vi "live_edited.vi"() -> ()   [LabVIEW 2020]
uses:
  C:/Users/Public/Documents/Photometrics/PMQI-LabViewSamples/Examples/2018/Dependencies/PVCamNET.dll
  Dependencies/PVCamNET.dll
panel:
  out "Trigger Mode":i32
  in  "Trigger In Behaviour":string(combo)
  out "Exp. out":i32
  in  "Trigger Out Behaviour":string(combo)
  out "Boolean":bool
  in  "Scan Direction Reset":bool
  out "Scan Line Time":dbl format="%#_14g"
  in  "Scan Width":dbl
  in  "Scan Line Delay":dbl
  in  "Scan Direction":string(combo)
  in  "Scan Mode":string(combo)
  in  "Exposure Time":dbl
  in  "Live":bool
  in  "Camera Status":bool
  in  "Uninit":bool
  in  "Live stop":bool
  in  "Live start":bool
  in  "Open":bool
  # "SimpleLiveAppProgrammableScanMode.vi\n\nDescription:\nThis sample code lets the user use programmable scan\n mode in an event driven structure.\n\nSteps to run:\n1. Click \"Run\"\n2. Click \"Open\"\n3. Enter Exposure Time\n4. Select Scan Mode. \n5. Set Scan Line Delay or Scan Width\n6. Select Scan Direction\n7. Click \"Live start\"\n8. Click \"Live stop\"\n9. Click \"Close\""
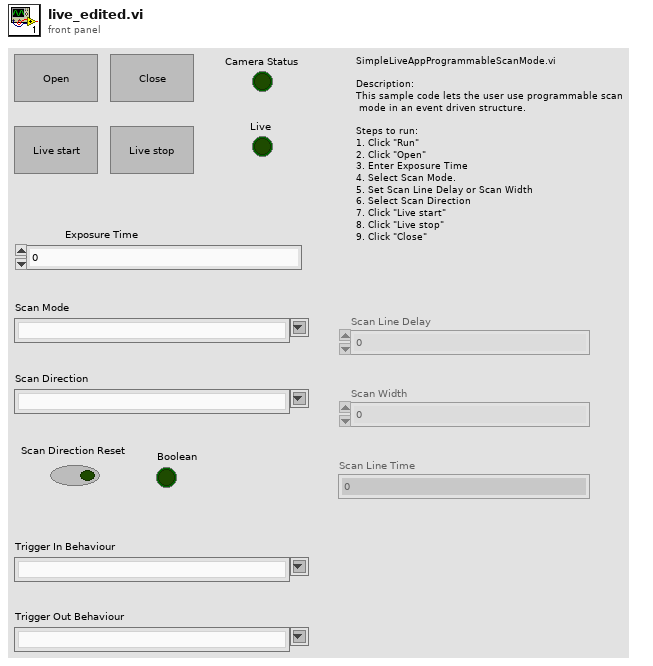
[diagram p1: front panel]
types:
  T1 = enum8{"Enabled", "Disabled", "Disabled and Grayed Out"}
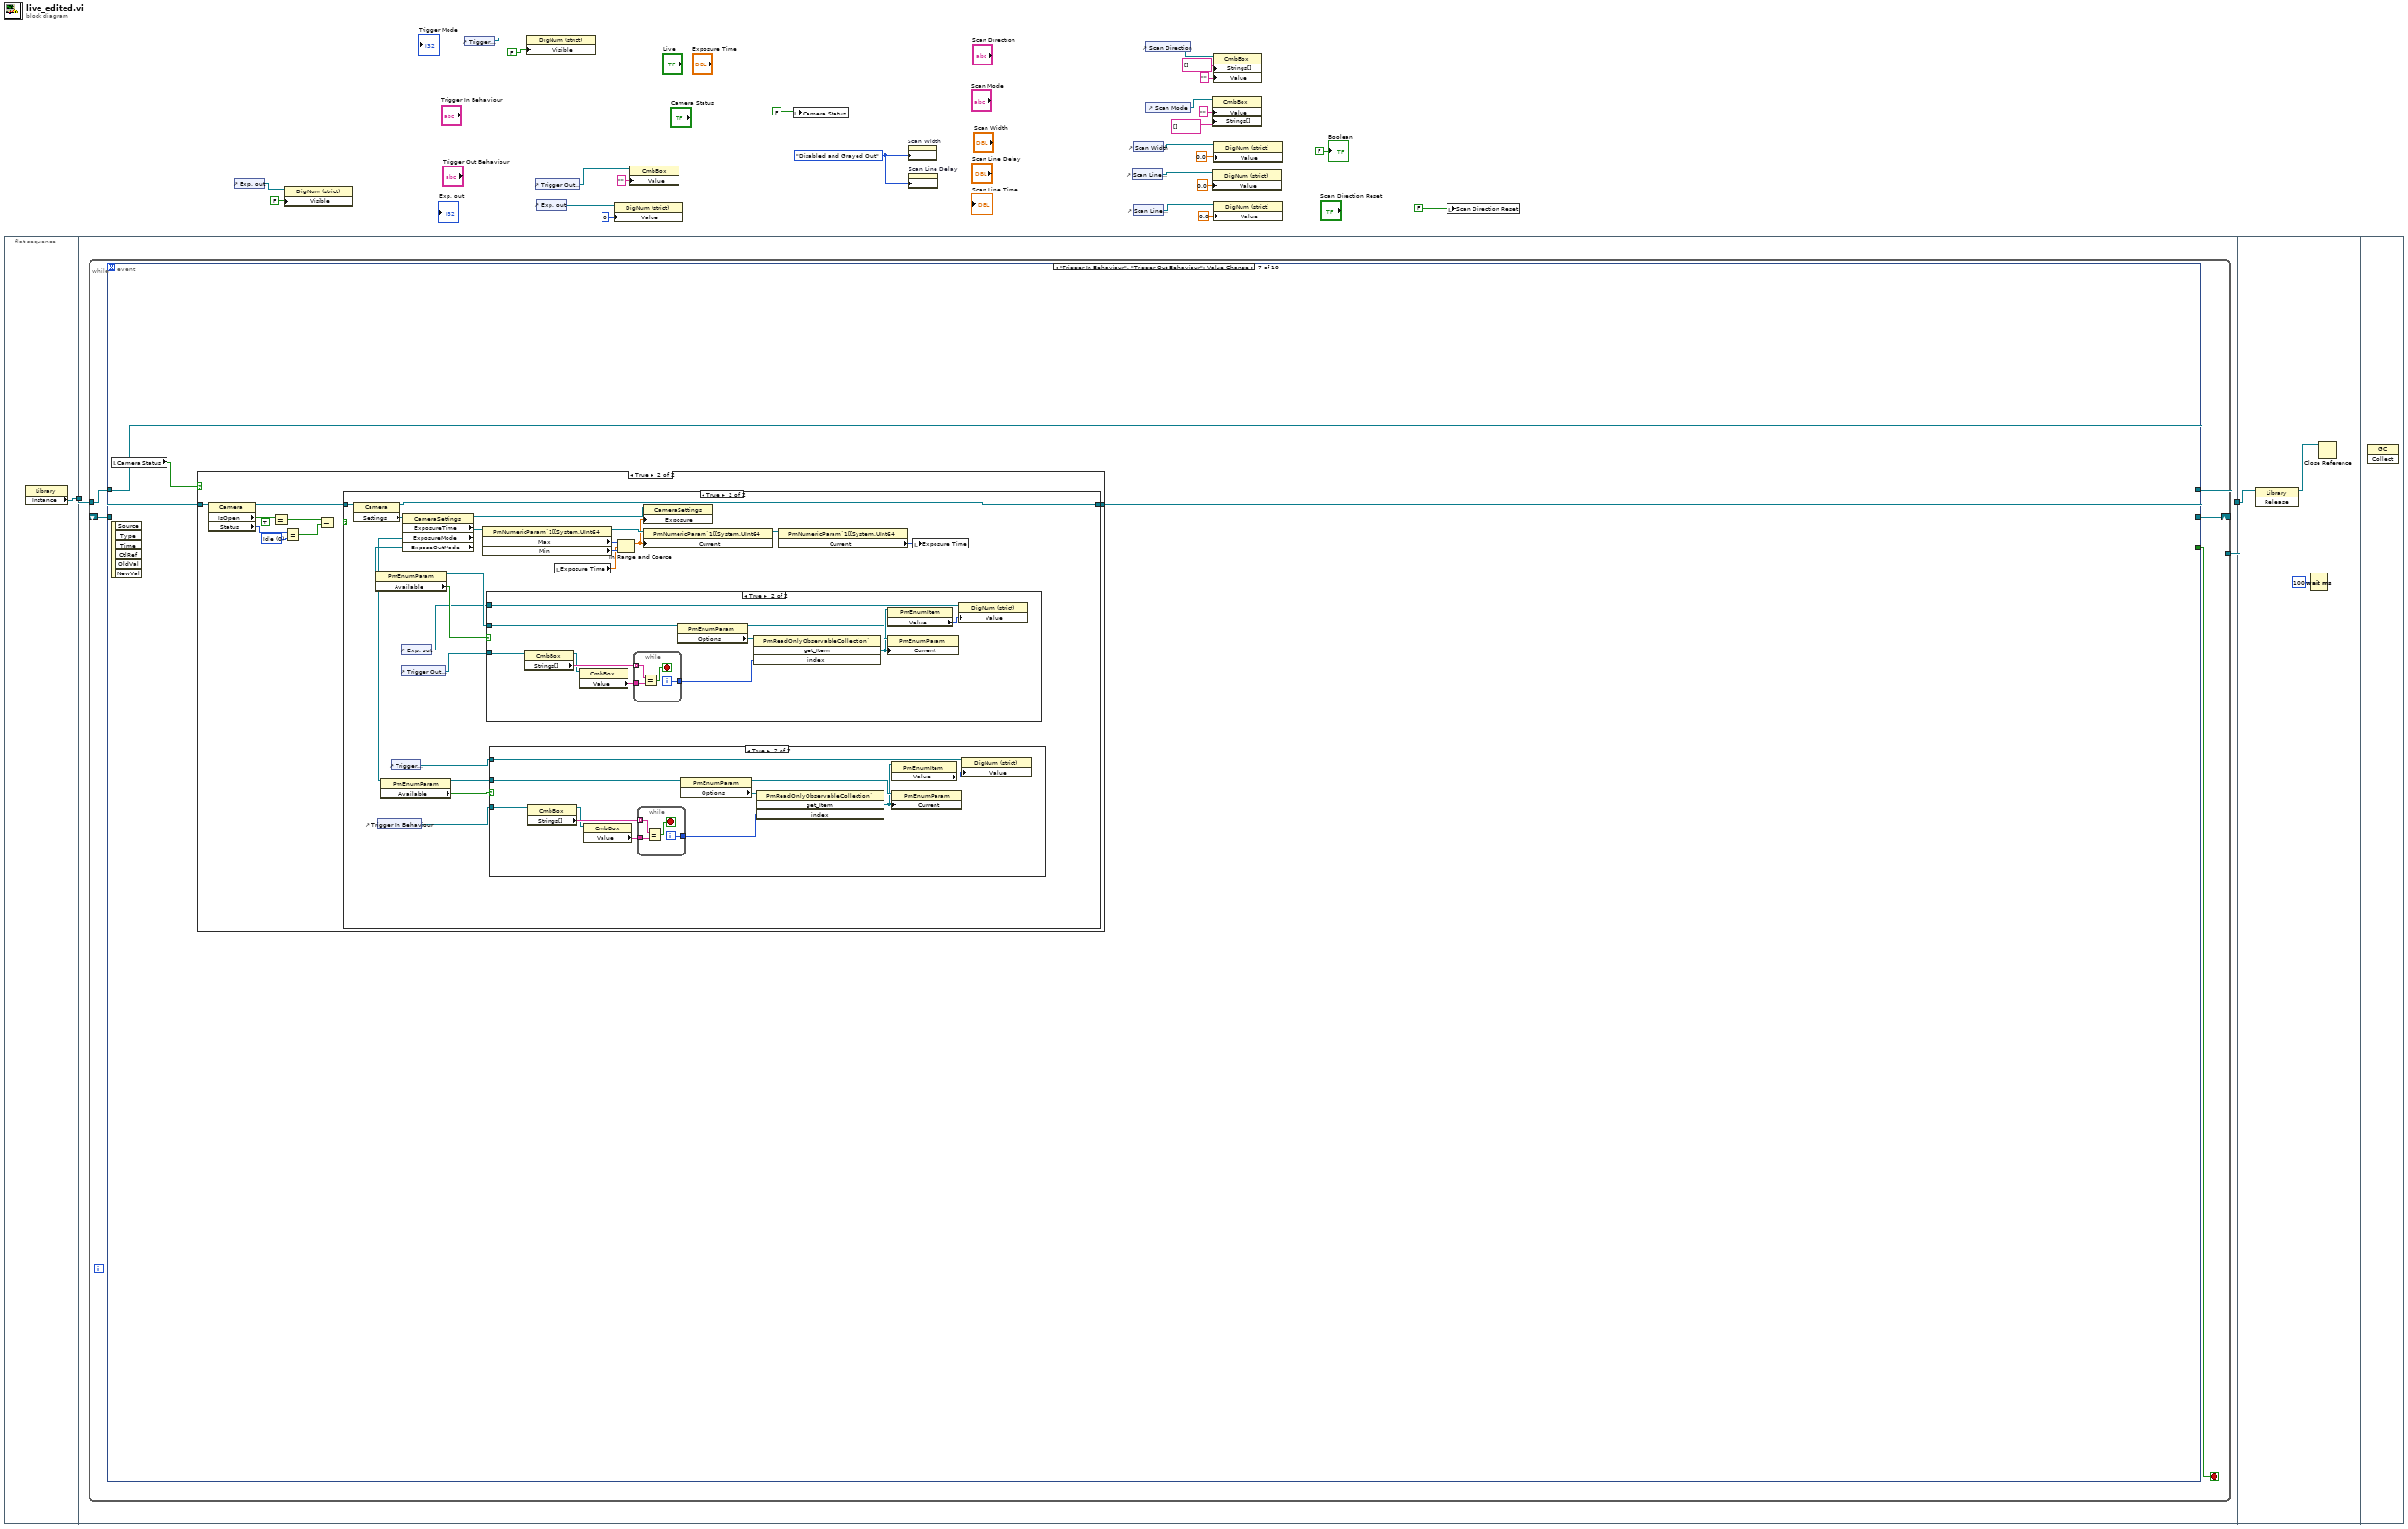
[diagram p0: block diagram]
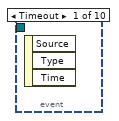
[diagram p2: hidden frame]
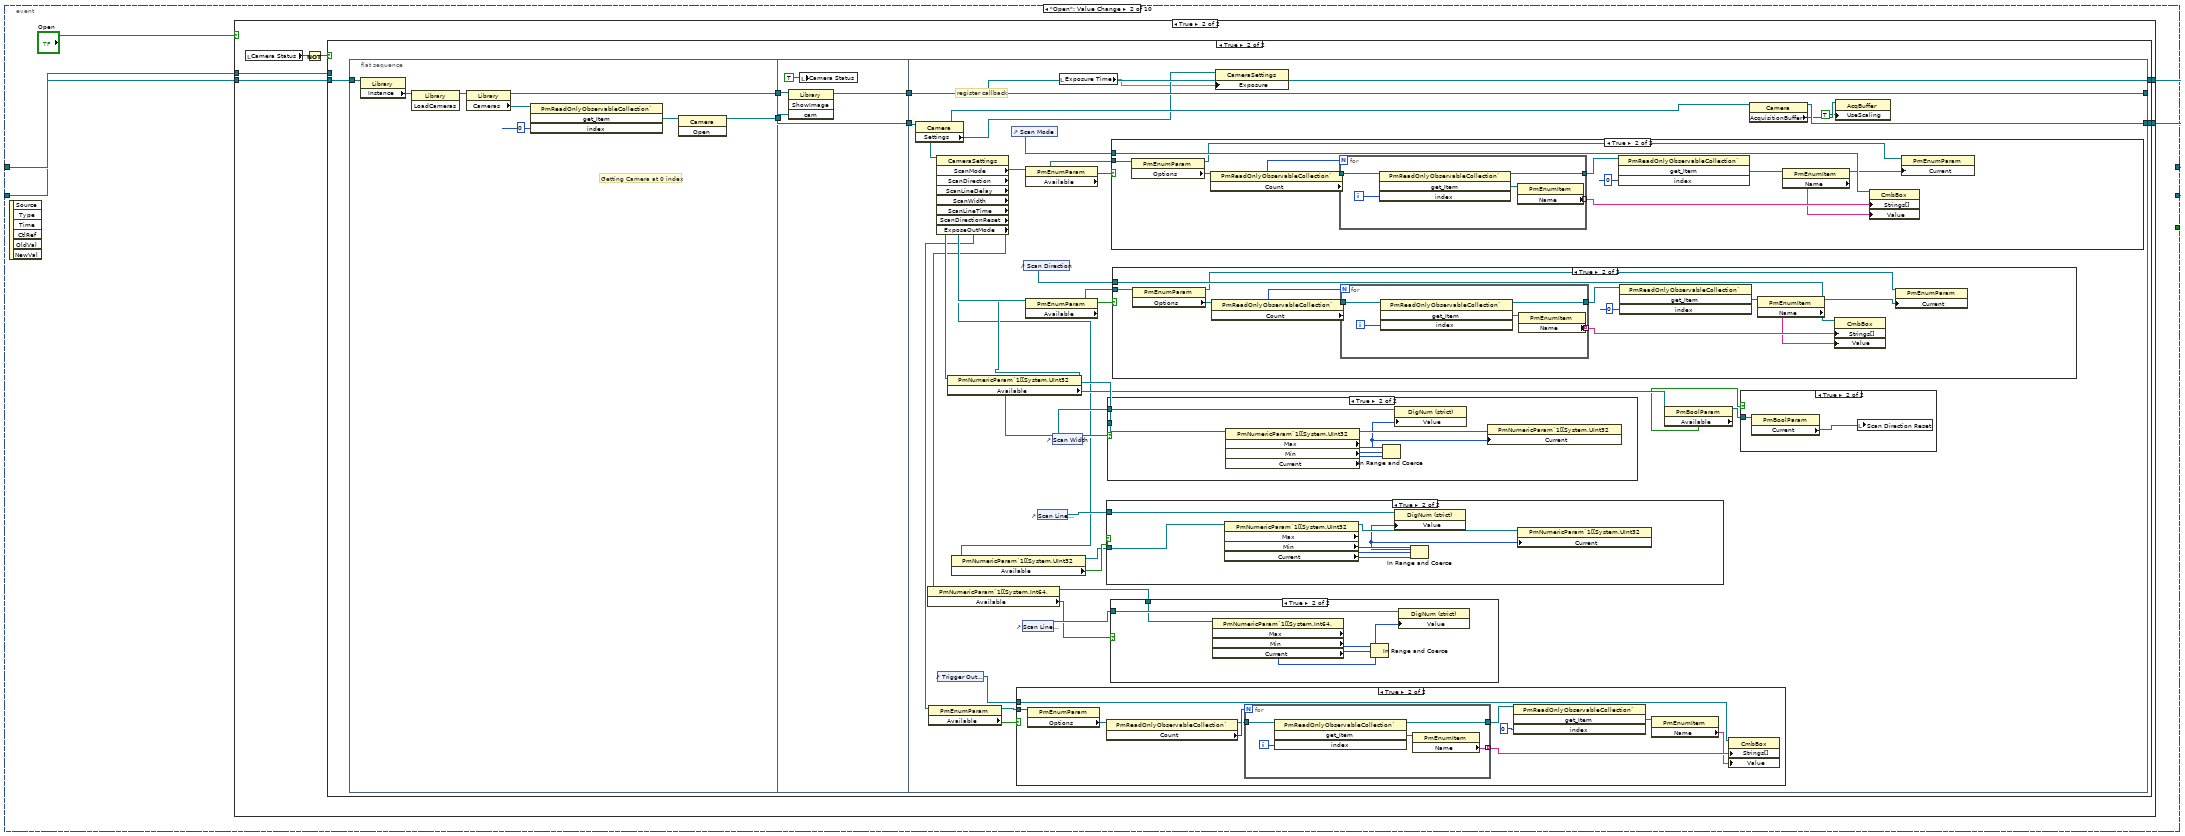
[diagram p3: hidden frame]
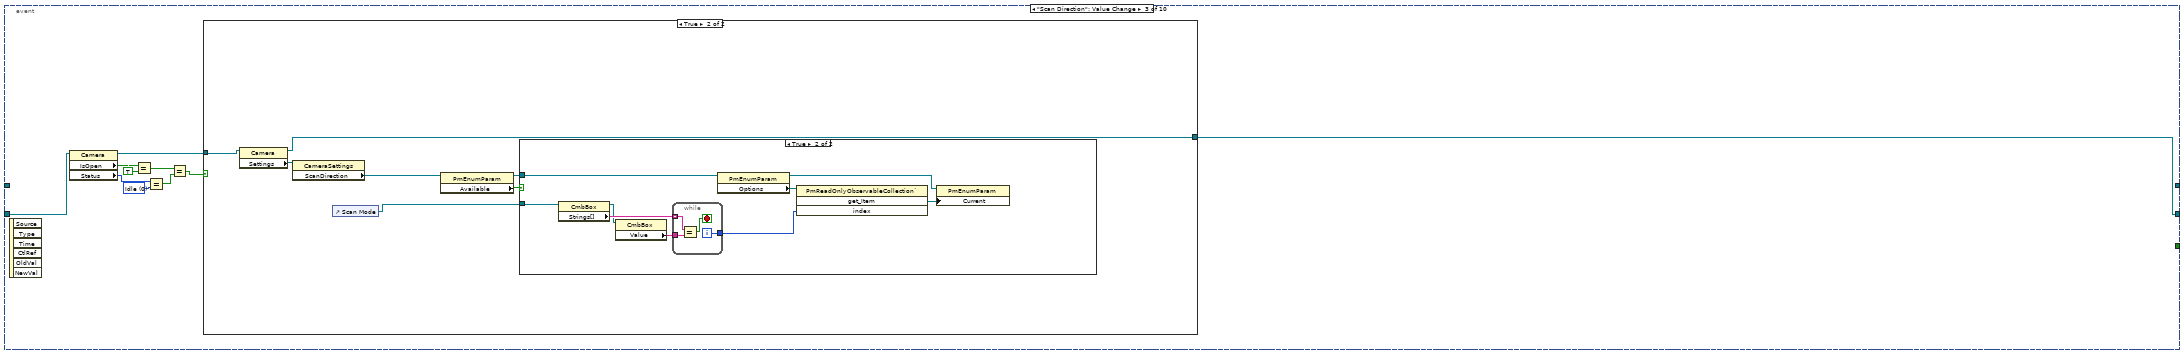
[diagram p13: hidden frame]
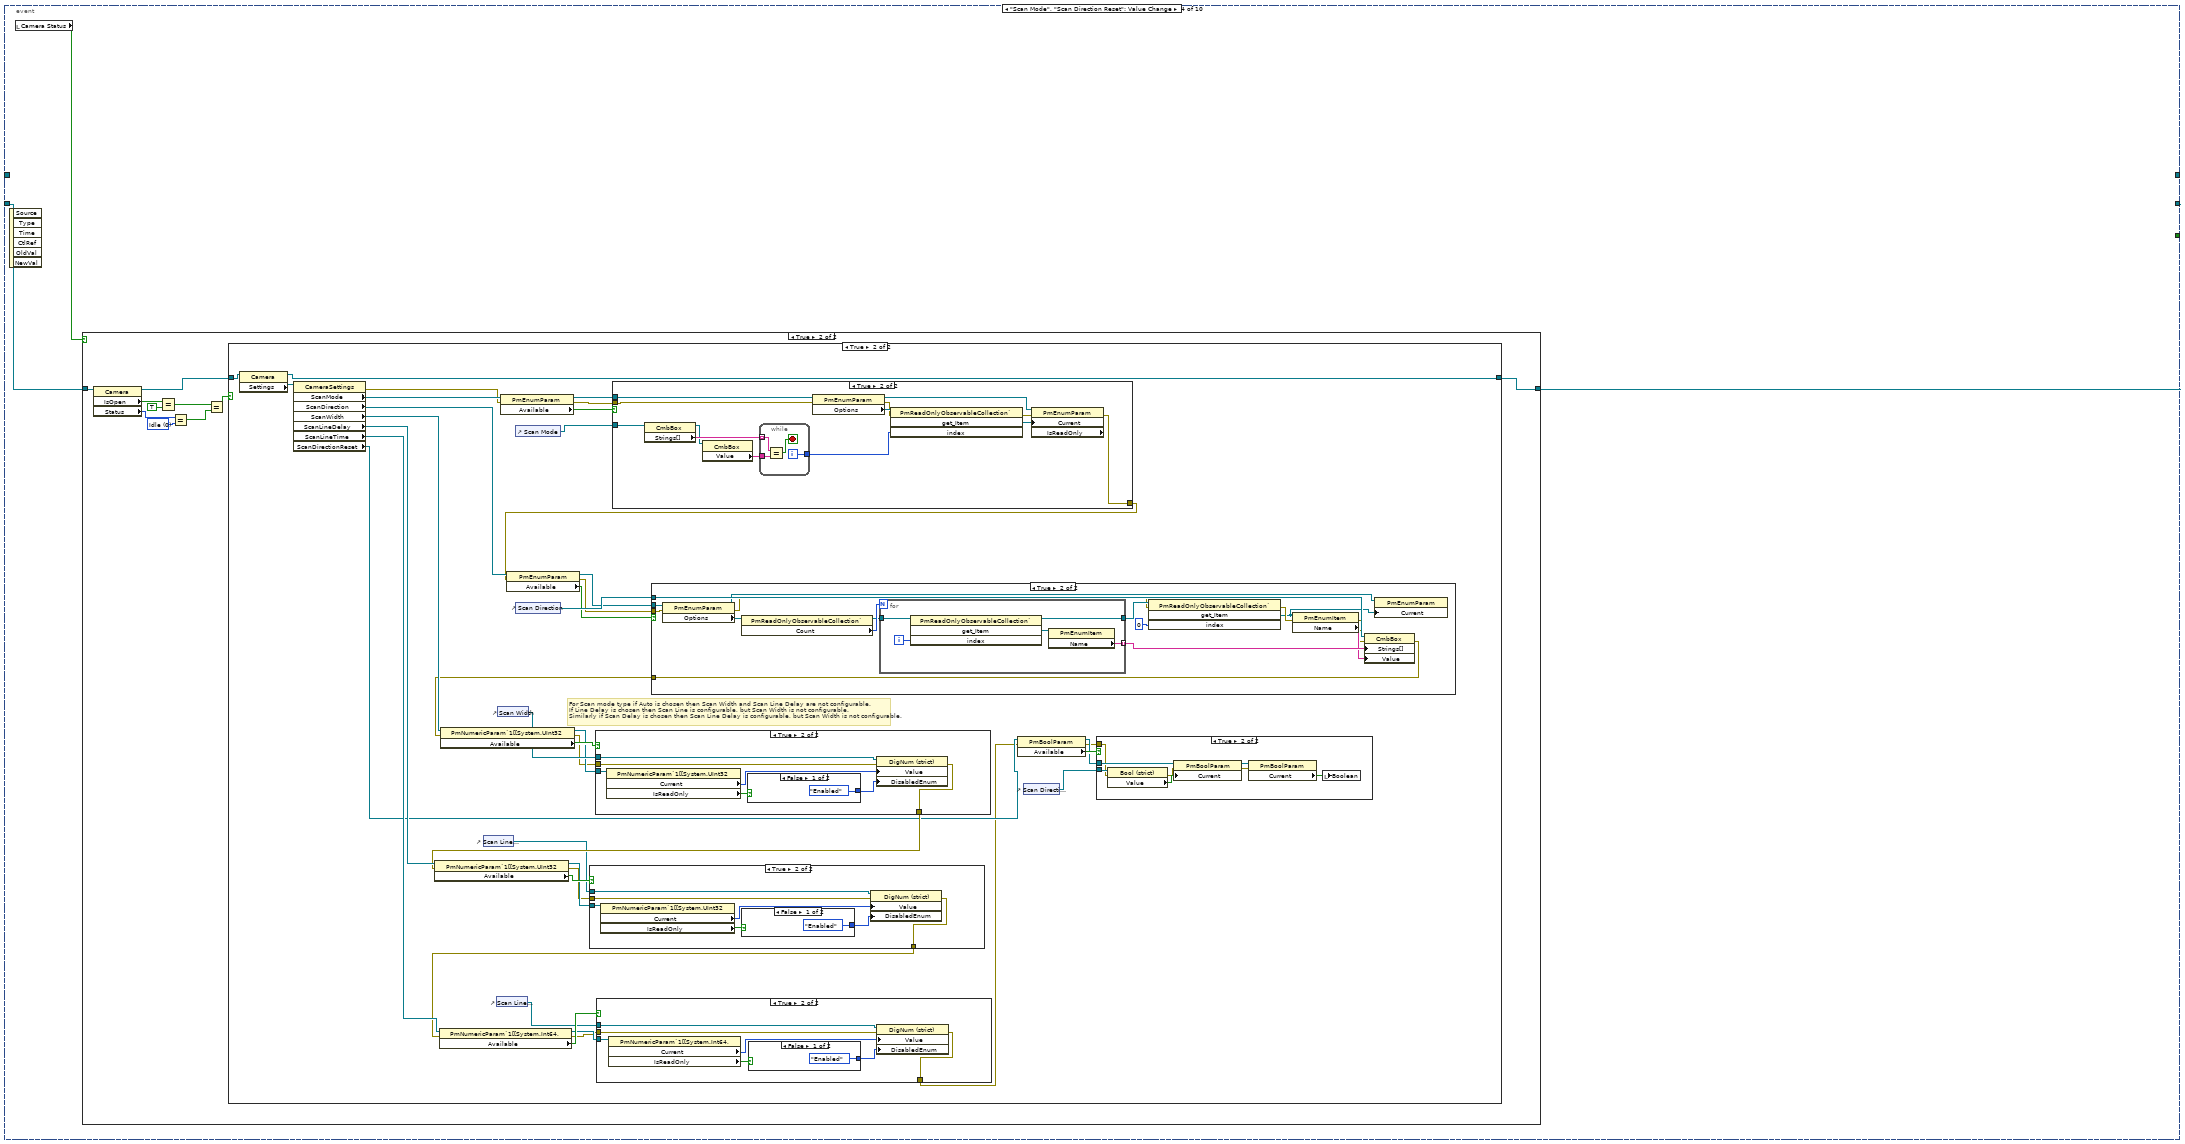
[diagram p16: hidden frame]
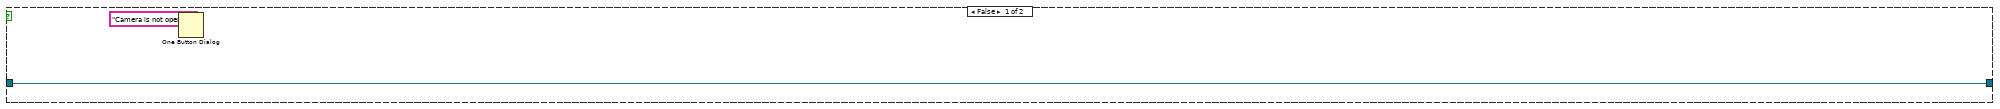
[diagram p17: hidden frame]
diagram:
  w11 = T1."Disabled and Grayed Out" ("Disabled")
  n1 = flat-sequence {
    tunnel: [w27] -> w26
    tunnel: w26 -> [w29]
    tunnel: [w28] -> w25
    tunnel: w25 -> [w613]
    frame #0 {
      n2 = property class="Library"() -> ("Instance"=w27:refnum<k24>)  [unwired: 2 in, 2 out]
    }
    frame #1 {
      n3 = while {
        tunnel: w29 -> [w34]
        shift-right: [w33] -> _
        shift-left: _ -> [w31]
        tunnel: [w32] -> w28
        stop <- w30 stop-if-true
        n4 = event shown="[6] \"Trigger In Behaviour\", \"Trigger Out Behaviour\": Value Change" {
          selector: _ -> [_ _ _ _ _ _ _ _ _ _]
          dyn-events: _ -> [_ _ _ _ _ _ _ _ _ _]
          timeout: _ -> [_ _ _ _ _ _ _ _ _ _]
          tunnel: w34 -> [_ w39 _ _ _ _ w462 w530 _ w585]
          tunnel: [_ w38 w175 w207 w339 w403 w463 w531 w560 w586] -> w33
          tunnel: [_ w37 _ _ _ _ w462 w530 _ w585] -> w32
          tunnel: w31 -> [_ w36 w179 w208 w345 w405 w464 w532 w561 w587]
          tunnel: [_ _ _ _ _ _ _ _ _ w584] -> w30
          event Timeout {
            n5 = event-data() -> ()  [unwired: 1 in, 3 out]
          }
          event "Open": Value Change {
            n6 = event-data() -> ()  [unwired: 1 in, 6 out]
            n7 = case shown="True" "Open" {
              tunnel: w39 -> [w41 w47]
              tunnel: [w40 w46] -> w38
              tunnel: [w41 w45] -> w37
              tunnel: w36 -> [w40 w42]
              frame False {
              }
              frame True {
                n8 = local read "Camera Status"() -> (w44:bool)
                n9 = Not(x=w44) -> (.not. x?=w43:bool)
                n10 = case shown="True" w43 {
                  tunnel: w47 -> [w48 w54]
                  tunnel: [w49 w53] -> w46
                  tunnel: [w48 w52] -> w45
                  tunnel: w42 -> [w49 _]
                  frame False {
                  }
                  frame True {
                    n11 = flat-sequence {
                      tunnel: w54 -> [w59]
                      tunnel: [w61] -> w56
                      tunnel: [w60] -> w55
                      tunnel: w56 -> [w67]
                      tunnel: w55 -> [w68]
                      tunnel: [w68] -> w51
                      tunnel: [w66] -> w50
                      tunnel: [w103] -> w52
                      tunnel: [w83] -> w53
                      tunnel: w51 -> [w102]
                      tunnel: w50 -> [w103]
                      frame #0 {
                        # "Getting Camera at 0 index"
                        n12 = property class="Library"(reference=w59) -> ("Instance"=w58:refnum<k24>)  [unwired: 1 in, 2 out]
                        n13 = invoke class="Library" method="LoadCameras"(reference=w58) -> (reference out=w57:refnum<k24>)  [unwired: 2 in, 2 out]
                        n14 = property class="Library"(reference=w57) -> (reference out=w61:refnum<k24>, "Cameras"=w64:refnum<k24>)  [unwired: 1 in, 1 out]
                        n15 = invoke class="PmReadOnlyObservableCollection`" method="get_Item"(reference=w64, "index"=0) -> ("get_Item"=w62:refnum<k24>)  [unwired: 2 in, 3 out]
                        n16 = invoke class="Camera" method="Open"(reference=w62) -> (reference out=w60:refnum<k24>)  [unwired: 2 in, 2 out]
                      }
                      frame #1 {
                        n17 = invoke class="Library" method="ShowImage"(reference=w67, "cam"=w68) -> (reference out=w66:refnum<k24>)  [unwired: 2 in, 3 out]
                        n18 = local write "Camera Status"(TRUE ("Camera Status")) -> ()
                      }
                      frame #2 {
                        # "register callback"
                        n19 = property class="Camera"(reference=w102) -> (reference out=w84:refnum<k24>, "Settings"=w73:refnum<k24>)  [unwired: 1 in, 1 out]
                        n20 = property class="CameraSettings"(reference=w73) -> ("ScanMode"=w101:refnum<k24>, "ScanDirection"=w97:refnum<k24>, "ScanLineDelay"=w92:refnum<k24>, "ScanWidth"=w79:refnum<k24>, "ScanLineTime"=w71:refnum<k24>, "ScanDirectionReset"=w87:refnum<k24>, "ExposeOutMode"=w75:refnum<k24>)  [unwired: 1 in, 2 out]
                        n21 = property class="PmNumericParam`1[[System.Int64,"(reference=w71) -> (reference out=w69:refnum<k24>, "Available"=w70:bool)  [unwired: 1 in, 1 out]
                        n22 = property class="PmEnumParam"(reference=w75) -> (reference out=w76:refnum<k24>, "Available"=w77:bool)  [unwired: 1 in, 1 out]
                        n23 = control-ref of="Trigger Out Behaviour"() -> (w74:refnum<vi>)
                        n24 = property class="PmNumericParam`1[[System.UInt32"(reference=w92) -> (reference out=w90:refnum<k24>, "Available"=w91:bool)  [unwired: 1 in, 1 out]
                        n25 = property class="PmNumericParam`1[[System.UInt32"(reference=w79) -> (reference out=w78:refnum<k24>, "Available"=w80:bool)  [unwired: 1 in, 1 out]
                        n26 = control-ref of="Scan Mode"() -> (w98:refnum<vi>)
                        n27 = case shown="True" w77 {
                          tunnel: w76 -> [_ w113]
                          tunnel: w74 -> [_ w104]
                          frame False {
                          }
                          frame True {
                            n28 = property class="PmEnumParam"(reference=w113) -> ("Options"=w112:refnum<k24>)  [unwired: 1 in, 2 out]
                            n29 = property class="PmReadOnlyObservableCollection`"(reference=w112) -> (reference out=w110:refnum<k24>, "Count"=w111:i32)  [unwired: 1 in, 1 out]
                            n30 = for {
                              N: w111 -> [_]
                              tunnel: w110 -> [w118]
                              tunnel: [w115] -> w107
                              tunnel: [w114] -> w106 mode=indexing
                              i -> [w117]
                              n31 = invoke class="PmReadOnlyObservableCollection`" method="get_Item"(reference=w118, "index"=w117) -> (reference out=w115:refnum<k24>, "get_Item"=w116:refnum<k24>)  [unwired: 2 in, 2 out]
                              n32 = property class="PmEnumItem"(reference=w116) -> ("Name"=w114:string)  [unwired: 1 in, 2 out]
                            }
                            n33 = invoke class="PmReadOnlyObservableCollection`" method="get_Item"(reference=w107, "index"=0) -> ("get_Item"=w108:refnum<k24>)  [unwired: 2 in, 3 out]
                            n34 = property class="PmEnumItem"(reference=w108) -> ("Name"=w105:string)  [unwired: 1 in, 2 out]
                            n35 = property class="CmbBox"(reference=w104, "Strings[]"=w106, "Value"=w105) -> ()  [unwired: 1 in, 2 out]
                          }
                        }
                        n36 = control-ref of="Scan Line Time"() -> (w88:refnum<vi>)
                        n37 = control-ref of="Scan Direction"() -> (w94:refnum<vi>)
                        n38 = property class="PmEnumParam"(reference=w101) -> (reference out=w99:refnum<k24>, "Available"=w100:bool)  [unwired: 1 in, 1 out]
                        n39 = property class="PmEnumParam"(reference=w97) -> (reference out=w95:refnum<k24>, "Available"=w96:bool)  [unwired: 1 in, 1 out]
                        n40 = control-ref of="Scan Line Delay"() -> (w89:refnum<vi>)
                        n41 = control-ref of="Scan Width"() -> (w93:refnum<vi>)
                        n42 = local read "Exposure Time"() -> (w72:dbl)
                        n43 = case shown="True" w80 {
                          tunnel: w89 -> [_ w130]
                          tunnel: w78 -> [_ w129]
                          frame False {
                          }
                          frame True {
                            n44 = property class="PmNumericParam`1[[System.UInt32"(reference=w129) -> (reference out=w128:refnum<k24>, "Max"=w131:u32, "Min"=w132:u32, "Current"=w133:u32)  [unwired: 1 in, 1 out]
                            n45 = In Range and Coerce(upper limit=w131, x=w133, lower limit=w132) -> (coerced(x)=w127:u32)  [unwired: 1 out]
                            n46 = property class="DigNum (strict)"(reference=w130, "Value"=w127) -> ()  [unwired: 1 in, 2 out]
                            n47 = property class="PmNumericParam`1[[System.UInt32"(reference=w128, "Current"=w127) -> ()  [unwired: 1 in, 2 out]
                          }
                        }
                        n48 = case shown="True" w91 {
                          tunnel: w93 -> [_ w137]
                          tunnel: w90 -> [_ w136]
                          frame False {
                          }
                          frame True {
                            n49 = property class="PmNumericParam`1[[System.UInt32"(reference=w136) -> (reference out=w135:refnum<k24>, "Max"=w138:u32, "Min"=w139:u32, "Current"=w140:u32)  [unwired: 1 in, 1 out]
                            n50 = In Range and Coerce(upper limit=w138, x=w140, lower limit=w139) -> (coerced(x)=w134:u32)  [unwired: 1 out]
                            n51 = property class="DigNum (strict)"(reference=w137, "Value"=w134) -> ()  [unwired: 1 in, 2 out]
                            n52 = property class="PmNumericParam`1[[System.UInt32"(reference=w135, "Current"=w134) -> ()  [unwired: 1 in, 2 out]
                          }
                        }
                        n53 = case shown="True" w70 {
                          tunnel: w88 -> [_ w122]
                          tunnel: w69 -> [_ w121]
                          frame False {
                          }
                          frame True {
                            n54 = property class="PmNumericParam`1[[System.Int64,"(reference=w121) -> ("Max"=w123:i64, "Min"=w124:i64, "Current"=w125:i64)  [unwired: 1 in, 2 out]
                            n55 = In Range and Coerce(upper limit=w123, x=w125, lower limit=w124) -> (coerced(x)=w126:i64)  [unwired: 1 out]
                            n56 = property class="DigNum (strict)"(reference=w122, "Value"=w126) -> ()  [unwired: 1 in, 2 out]
                          }
                        }
                        n57 = case shown="True" w100 {
                          tunnel: w99 -> [_ w169]
                          tunnel: w98 -> [_ w161]
                          frame False {
                          }
                          frame True {
                            n58 = property class="PmEnumParam"(reference=w169) -> (reference out=w160:refnum<k24>, "Options"=w168:refnum<k24>)  [unwired: 1 in, 1 out]
                            n59 = property class="PmReadOnlyObservableCollection`"(reference=w168) -> (reference out=w166:refnum<k24>, "Count"=w167:i32)  [unwired: 1 in, 1 out]
                            n60 = for {
                              N: w167 -> [_]
                              tunnel: w166 -> [w174]
                              tunnel: [w171] -> w164
                              tunnel: [w170] -> w163 mode=indexing
                              i -> [w173]
                              n61 = invoke class="PmReadOnlyObservableCollection`" method="get_Item"(reference=w174, "index"=w173) -> (reference out=w171:refnum<k24>, "get_Item"=w172:refnum<k24>)  [unwired: 2 in, 2 out]
                              n62 = property class="PmEnumItem"(reference=w172) -> ("Name"=w170:string)  [unwired: 1 in, 2 out]
                            }
                            n63 = invoke class="PmReadOnlyObservableCollection`" method="get_Item"(reference=w164, "index"=0) -> ("get_Item"=w159:refnum<k24>)  [unwired: 2 in, 3 out]
                            n64 = property class="PmEnumItem"(reference=w159) -> (reference out=w158:refnum<k24>, "Name"=w162:string)  [unwired: 1 in, 1 out]
                            n65 = property class="CmbBox"(reference=w161, "Strings[]"=w163, "Value"=w162) -> ()  [unwired: 1 in, 2 out]
                            n66 = property class="PmEnumParam"(reference=w160, "Current"=w158) -> ()  [unwired: 1 in, 2 out]
                          }
                        }
                        n67 = case shown="True" w96 {
                          tunnel: w95 -> [_ w152]
                          tunnel: w94 -> [_ w143]
                          frame False {
                          }
                          frame True {
                            n68 = property class="PmEnumParam"(reference=w152) -> (reference out=w142:refnum<k24>, "Options"=w151:refnum<k24>)  [unwired: 1 in, 1 out]
                            n69 = property class="PmReadOnlyObservableCollection`"(reference=w151) -> (reference out=w149:refnum<k24>, "Count"=w150:i32)  [unwired: 1 in, 1 out]
                            n70 = for {
                              N: w150 -> [_]
                              tunnel: w149 -> [w157]
                              tunnel: [w154] -> w146
                              tunnel: [w153] -> w145 mode=indexing
                              i -> [w156]
                              n71 = invoke class="PmReadOnlyObservableCollection`" method="get_Item"(reference=w157, "index"=w156) -> (reference out=w154:refnum<k24>, "get_Item"=w155:refnum<k24>)  [unwired: 2 in, 2 out]
                              n72 = property class="PmEnumItem"(reference=w155) -> ("Name"=w153:string)  [unwired: 1 in, 2 out]
                            }
                            n73 = invoke class="PmReadOnlyObservableCollection`" method="get_Item"(reference=w146, "index"=0) -> ("get_Item"=w147:refnum<k24>)  [unwired: 2 in, 3 out]
                            n74 = property class="PmEnumItem"(reference=w147) -> (reference out=w141:refnum<k24>, "Name"=w144:string)  [unwired: 1 in, 1 out]
                            n75 = property class="CmbBox"(reference=w143, "Strings[]"=w145, "Value"=w144) -> ()  [unwired: 1 in, 2 out]
                            n76 = property class="PmEnumParam"(reference=w142, "Current"=w141) -> ()  [unwired: 1 in, 2 out]
                          }
                        }
                        n77 = property class="CameraSettings"(reference=w73, "Exposure"=w72) -> ()  [unwired: 1 in, 2 out]
                        n78 = property class="PmBoolParam"(reference=w87) -> (reference out=w85:refnum<k24>, "Available"=w86:bool)  [unwired: 1 in, 1 out]
                        n79 = case shown="True" w86 {
                          tunnel: w85 -> [_ w120]
                          frame False {
                          }
                          frame True {
                            n80 = property class="PmBoolParam"(reference=w120) -> ("Current"=w119:bool)  [unwired: 1 in, 2 out]
                            n81 = local write "Scan Direction Reset"(w119) -> ()
                          }
                        }
                        n82 = property class="Camera"(reference=w84) -> (reference out=w83:refnum<k24>, "AcquisitionBuffer"=w82:refnum<k24>)  [unwired: 1 in, 1 out]
                        n83 = property class="AcqBuffer"(reference=w82, "UseScaling"=TRUE) -> ()  [unwired: 1 in, 2 out]
                      }
                    }
                  }
                }
              }
            }
          }
          event "Scan Direction": Value Change {
            w183 = 0 items=["Idle", "Capturing"] ("Status")
            n84 = event-data() -> ()  [unwired: 1 in, 6 out]
            n85 = property class="Camera"(reference=w179) -> (reference out=w176:refnum<k24>, "IsOpen"=w182:bool, "Status"=w184:i32)  [unwired: 1 in, 1 out]
            n86 = Equal?(x=w182, y=TRUE) -> (x = y?=w178:bool)
            n87 = Equal?(x=w184, y=w183) -> (x = y?=w180:bool)
            n88 = Equal?(x=w178, y=w180) -> (x = y?=w177:bool)
            n89 = case shown="True" w177 {
              tunnel: w176 -> [w185 w189]
              tunnel: [w185 w186] -> w175
              frame False {
              }
              frame True {
                n90 = property class="Camera"(reference=w189) -> (reference out=w186:refnum<k24>, "Settings"=w190:refnum<k24>)  [unwired: 1 in, 1 out]
                n91 = property class="CameraSettings"(reference=w190) -> ("ScanDirection"=w188:refnum<k24>)  [unwired: 1 in, 2 out]
                n92 = control-ref of="Scan Mode"() -> (w187:refnum<vi>)
                n93 = property class="PmEnumParam"(reference=w188) -> (reference out=w191:refnum<k24>, "Available"=w192:bool)  [unwired: 1 in, 1 out]
                n94 = case shown="True" w192 {
                  tunnel: w191 -> [_ w200]
                  tunnel: w187 -> [_ w193]
                  frame False {
                  }
                  frame True {
                    n95 = property class="CmbBox"(reference=w193) -> (reference out=w195:refnum<vi>, "Strings[]"=w201:string[])  [unwired: 1 in, 1 out]
                    n96 = property class="CmbBox"(reference=w195) -> ("Value"=w194:string)  [unwired: 1 in, 2 out]
                    n97 = while {
                      tunnel: w201 -> [w205] mode=indexing
                      tunnel: [w203] -> w198
                      tunnel: w194 -> [w202]
                      i -> [w203]
                      stop <- w204 stop-if-true
                      n98 = Equal?(x=w205, y=w202) -> (x = y?=w204:bool)
                    }
                    n99 = property class="PmEnumParam"(reference=w200) -> (reference out=w197:refnum<k24>, "Options"=w199:refnum<k24>)  [unwired: 1 in, 1 out]
                    n100 = invoke class="PmReadOnlyObservableCollection`" method="get_Item"(reference=w199, "index"=w198) -> ("get_Item"=w196:refnum<k24>)  [unwired: 2 in, 3 out]
                    n101 = property class="PmEnumParam"(reference=w197, "Current"=w196) -> ()  [unwired: 1 in, 2 out]
                  }
                }
              }
            }
          }
          event "Scan Mode", "Scan Direction Reset": Value Change {
            n102 = event-data() -> ()  [unwired: 1 in, 6 out]
            n103 = local read "Camera Status"() -> (w206:bool)
            n104 = case shown="True" w206 {
              tunnel: w208 -> [w209 w214]
              tunnel: [w209 w212] -> w207
              frame False {
                n105 = One Button Dialog(message="Camera is not open") -> ()  [unwired: 1 in, 1 out]
              }
              frame True {
                w219 = 0 items=["Idle", "Capturing"] ("Status")
                n106 = property class="Camera"(reference=w214) -> (reference out=w213:refnum<k24>, "IsOpen"=w218:bool, "Status"=w220:i32)  [unwired: 1 in, 1 out]
                n107 = Equal?(x=w218, y=TRUE) -> (x = y?=w216:bool)
                n108 = Equal?(x=w220, y=w219) -> (x = y?=w215:bool)
                n109 = Equal?(x=w216, y=w215) -> (x = y?=w211:bool)
                n110 = case shown="True" w211 {
                  tunnel: w213 -> [w221 w260]
                  tunnel: [w221 w255] -> w212
                  frame False {
                  }
                  frame True {
                    # "For Scan mode type if Auto is chosen then Scan Width and Scan Line Delay are not configurable.\nIf Line Delay is chosen then Scan Line is configurable, but Scan Width is not configurable.\nSimilarly if Scan Delay is chosen then Scan Line Delay is configurable, but Scan Width is not configurable."
                    n111 = property class="Camera"(reference=w260) -> (reference out=w255:refnum<k24>, "Settings"=w259:refnum<k24>)  [unwired: 1 in, 1 out]
                    n112 = property class="CameraSettings"(reference=w259) -> (error out=w252:errorcluster, "ScanMode"=w258:refnum<k24>, "ScanDirection"=w254:refnum<k24>, "ScanWidth"=w250:refnum<k24>, "ScanLineDelay"=w249:refnum<k24>, "ScanLineTime"=w238:refnum<k24>, "ScanDirectionReset"=w227:refnum<k24>)  [unwired: 1 in, 1 out]
                    n113 = control-ref of="Scan Line Delay"() -> (w229:refnum<vi>)
                    n114 = control-ref of="Scan Line Time"() -> (w232:refnum<vi>)
                    n115 = control-ref of="Scan Width"() -> (w245:refnum<vi>)
                    n116 = property class="PmEnumParam"(reference=w258, error in=w252) -> (reference out=w256:refnum<k24>, error out=w253:errorcluster, "Available"=w257:bool)
                    n117 = control-ref of="Scan Mode"() -> (w251:refnum<vi>)
                    n118 = control-ref of="Scan Direction"() -> (w248:refnum<vi>)
                    n119 = case shown="True" w257 {
                      tunnel: w256 -> [_ w333]
                      tunnel: w251 -> [_ w328]
                      tunnel: w253 -> [w321 w327]
                      tunnel: [w321 w322] -> w237
                      frame False {
                      }
                      frame True {
                        n120 = property class="CmbBox"(reference=w328) -> (reference out=w329:refnum<vi>, "Strings[]"=w334:string[])  [unwired: 1 in, 1 out]
                        n121 = property class="CmbBox"(reference=w329) -> ("Value"=w324:string)  [unwired: 1 in, 2 out]
                        n122 = while {
                          tunnel: w334 -> [w338] mode=indexing
                          tunnel: [w336] -> w331
                          tunnel: w324 -> [w335]
                          i -> [w336]
                          stop <- w337 stop-if-true
                          n123 = Equal?(x=w338, y=w335) -> (x = y?=w337:bool)
                        }
                        n124 = property class="PmEnumParam"(reference=w333, error in=w327) -> (reference out=w330:refnum<k24>, error out=w326:errorcluster, "Options"=w332:refnum<k24>)
                        n125 = invoke class="PmReadOnlyObservableCollection`" method="get_Item"(reference=w332, error in=w326, "index"=w331) -> (error out=w325:errorcluster, "get_Item"=w323:refnum<k24>)  [unwired: 1 in, 2 out]
                        n126 = property class="PmEnumParam" props=["Current", "IsReadOnly"](reference=w330, error in=w325, "Current"=w323) -> (error out=w322:errorcluster)  [unwired: 2 out]
                      }
                    }
                    n127 = property class="PmEnumParam"(reference=w254, error in=w237) -> (reference out=w246:refnum<k24>, error out=w240:errorcluster, "Available"=w247:bool)
                    n128 = case shown="True" w247 {
                      tunnel: w246 -> [_ w315]
                      tunnel: w248 -> [_ w307]
                      tunnel: w240 -> [w299 w306]
                      tunnel: [w299 w300] -> w239
                      frame False {
                      }
                      frame True {
                        n129 = property class="PmEnumParam"(reference=w315, error in=w306) -> (reference out=w301:refnum<k24>, error out=w305:errorcluster, "Options"=w314:refnum<k24>)
                        n130 = property class="PmReadOnlyObservableCollection`"(reference=w314) -> (reference out=w312:refnum<k24>, "Count"=w313:i32)  [unwired: 1 in, 1 out]
                        n131 = for {
                          N: w313 -> [_]
                          tunnel: w312 -> [w320]
                          tunnel: [w317] -> w310
                          tunnel: [w316] -> w309 mode=indexing
                          i -> [w319]
                          n132 = invoke class="PmReadOnlyObservableCollection`" method="get_Item"(reference=w320, "index"=w319) -> (reference out=w317:refnum<k24>, "get_Item"=w318:refnum<k24>)  [unwired: 2 in, 2 out]
                          n133 = property class="PmEnumItem"(reference=w318) -> ("Name"=w316:string)  [unwired: 1 in, 2 out]
                        }
                        n134 = invoke class="PmReadOnlyObservableCollection`" method="get_Item"(reference=w310, error in=w305, "index"=0) -> (error out=w304:errorcluster, "get_Item"=w302:refnum<k24>)  [unwired: 1 in, 2 out]
                        n135 = property class="PmEnumItem"(reference=w302, error in=w304) -> (error out=w303:errorcluster, "Name"=w308:string)  [unwired: 1 out]
                        n136 = property class="CmbBox"(reference=w307, error in=w303, "Strings[]"=w309, "Value"=w308) -> (error out=w300:errorcluster)  [unwired: 1 out]
                        n137 = property class="PmEnumParam"(reference=w301, "Current"=w302) -> ()  [unwired: 1 in, 2 out]
                      }
                    }
                    n138 = property class="PmNumericParam`1[[System.UInt32"(reference=w250, error in=w239) -> (reference out=w243:refnum<k24>, error out=w242:errorcluster, "Available"=w244:bool)
                    n139 = case shown="True" w244 {
                      tunnel: w245 -> [_ w295]
                      tunnel: w243 -> [_ w292]
                      tunnel: w242 -> [w289 w294]
                      tunnel: [w289 w293] -> w241
                      frame False {
                      }
                      frame True {
                        n140 = property class="PmNumericParam`1[[System.UInt32"(reference=w292) -> ("Current"=w296:u32, "IsReadOnly"=w291:bool)  [unwired: 1 in, 2 out]
                        n141 = case shown="False" w291 {
                          tunnel: [T1."Enabled" ("Disabled") T1."Disabled and Grayed Out" ("Disabled")] -> w290
                          frame False {
                          }
                          frame True {
                          }
                        }
                        n142 = property class="DigNum (strict)"(reference=w295, error in=w294, "Value"=w296, "DisabledEnum"=w290) -> (error out=w293:errorcluster)  [unwired: 1 out]
                      }
                    }
                    n143 = property class="PmNumericParam`1[[System.UInt32"(reference=w249, error in=w241) -> (reference out=w234:refnum<k24>, error out=w228:errorcluster, "Available"=w235:bool)
                    n144 = case shown="True" w235 {
                      tunnel: w229 -> [_ w285]
                      tunnel: w234 -> [_ w282]
                      tunnel: w228 -> [w279 w284]
                      tunnel: [w279 w283] -> w231
                      frame False {
                      }
                      frame True {
                        n145 = property class="PmNumericParam`1[[System.UInt32"(reference=w282) -> ("Current"=w286:u32, "IsReadOnly"=w281:bool)  [unwired: 1 in, 2 out]
                        n146 = case shown="False" w281 {
                          tunnel: [T1."Enabled" ("Disabled") T1."Disabled and Grayed Out" ("Disabled")] -> w280
                          frame False {
                          }
                          frame True {
                          }
                        }
                        n147 = property class="DigNum (strict)"(reference=w285, error in=w284, "Value"=w286, "DisabledEnum"=w280) -> (error out=w283:errorcluster)  [unwired: 1 out]
                      }
                    }
                    n148 = property class="PmNumericParam`1[[System.Int64,"(reference=w238, error in=w231) -> (reference out=w233:refnum<k24>, error out=w230:errorcluster, "Available"=w236:bool)
                    n149 = case shown="True" w236 {
                      tunnel: w232 -> [_ w275]
                      tunnel: w233 -> [_ w272]
                      tunnel: w230 -> [w269 w274]
                      tunnel: [w269 w273] -> w223
                      frame False {
                      }
                      frame True {
                        n150 = property class="PmNumericParam`1[[System.Int64,"(reference=w272) -> ("Current"=w276:i64, "IsReadOnly"=w271:bool)  [unwired: 1 in, 2 out]
                        n151 = case shown="False" w271 {
                          tunnel: [T1."Enabled" ("Disabled") T1."Disabled and Grayed Out" ("Disabled")] -> w270
                          frame False {
                          }
                          frame True {
                          }
                        }
                        n152 = property class="DigNum (strict)"(reference=w275, error in=w274, "Value"=w276, "DisabledEnum"=w270) -> (error out=w273:errorcluster)  [unwired: 1 out]
                      }
                    }
                    n153 = property class="PmBoolParam"(reference=w227, error in=w223) -> (reference out=w225:refnum<k24>, error out=w222:errorcluster, "Available"=w226:bool)
                    n154 = control-ref of="Scan Direction Reset"() -> (w224:refnum<vi>)
                    n155 = case shown="True" w226 {
                      tunnel: w225 -> [_ w266]
                      tunnel: w224 -> [_ w268]
                      tunnel: w222 -> [_ w263]
                      frame False {
                      }
                      frame True {
                        n156 = property class="Bool (strict)"(reference=w268, error in=w263) -> (error out=w262:errorcluster, "Value"=w267:bool)  [unwired: 1 out]
                        n157 = property class="PmBoolParam"(reference=w266, error in=w262, "Current"=w267) -> (reference out=w265:refnum<k24>, error out=w261:errorcluster)
                        n158 = property class="PmBoolParam"(reference=w265, error in=w261) -> ("Current"=w264:bool)  [unwired: 2 out]
                        n159 = local write "Boolean"(w264) -> ()
                      }
                    }
                  }
                }
              }
            }
          }
          event "Scan Line Delay": Value Change {
            w350 = 0 items=["Idle", "Capturing"] ("Status")
            n160 = event-data() -> ()  [unwired: 1 in, 6 out]
            n161 = property class="Camera"(reference=w345) -> (reference out=w344:refnum<k24>, "IsOpen"=w349:bool, "Status"=w351:i32)  [unwired: 1 in, 1 out]
            n162 = Equal?(x=w349, y=TRUE) -> (x = y?=w347:bool)
            n163 = Equal?(x=w351, y=w350) -> (x = y?=w346:bool)
            n164 = Equal?(x=w347, y=w346) -> (x = y?=w343:bool)
            n165 = control-ref of="Scan Line Time"() -> (w340:refnum<vi>)
            n166 = control-ref of="Scan Line Delay"() -> (w341:refnum<vi>)
            n167 = control-ref of="Scan Width"() -> (w342:refnum<vi>)
            n168 = case shown="True" w343 {
              tunnel: w344 -> [w352 w374]
              tunnel: [w352 w373] -> w339
              tunnel: w341 -> [_ w372]
              tunnel: w342 -> [_ w371]
              tunnel: w340 -> [_ w355]
              frame False {
              }
              frame True {
                n169 = property class="Camera"(reference=w374) -> (reference out=w373:refnum<k24>, "Settings"=w370:refnum<k24>)  [unwired: 1 in, 1 out]
                n170 = property class="CameraSettings"(reference=w370) -> (reference out=w360:refnum<k24>, error out=w366:errorcluster, "ScanLineDelay"=w369:refnum<k24>)  [unwired: 1 in]
                n171 = property class="PmNumericParam`1[[System.UInt32"(reference=w369, error in=w366) -> (reference out=w367:refnum<k24>, error out=w365:errorcluster, "Available"=w368:bool)
                n172 = case shown="True" w368 {
                  tunnel: w372 -> [_ w391]
                  tunnel: w367 -> [_ w390]
                  tunnel: w365 -> [w386 w389]
                  tunnel: [w386 w387] -> w361
                  frame False {
                  }
                  frame True {
                    n173 = property class="PmNumericParam`1[[System.UInt32"(reference=w390) -> (reference out=w394:refnum<k24>, "Max"=w392:u32, "Min"=w393:u32)  [unwired: 1 in, 1 out]
                    n174 = property class="DigNum (strict)"(reference=w391, error in=w389) -> (reference out=w398:refnum<vi>, error out=w388:errorcluster, "Value"=w397:dbl)
                    n175 = In Range and Coerce(upper limit=w392, x=w397, lower limit=w393) -> (coerced(x)=w396:dbl)  [unwired: 1 out]
                    n176 = property class="PmNumericParam`1[[System.UInt32"(reference=w394, "Current"=w396) -> (reference out=w395:refnum<k24>)  [unwired: 1 in, 1 out]
                    n177 = property class="PmNumericParam`1[[System.UInt32"(reference=w395) -> ("Current"=w399:u32)  [unwired: 1 in, 2 out]
                    n178 = property class="DigNum (strict)"(reference=w398, error in=w388, "Value"=w399) -> (error out=w387:errorcluster)  [unwired: 1 out]
                  }
                }
                n179 = property class="CameraSettings"(reference=w360) -> ("ScanWidth"=w359:refnum<k24>, "ScanLineTime"=w358:refnum<k24>)  [unwired: 1 in, 2 out]
                n180 = property class="PmNumericParam`1[[System.UInt32"(reference=w359, error in=w361) -> (reference out=w363:refnum<k24>, error out=w362:errorcluster, "Available"=w364:bool)
                n181 = case shown="True" w364 {
                  tunnel: w371 -> [_ w382]
                  tunnel: w363 -> [_ w385]
                  tunnel: w362 -> [w380 w383]
                  tunnel: [w380 w384] -> w354
                  frame False {
                  }
                  frame True {
                    n182 = property class="PmNumericParam`1[[System.UInt32"(reference=w385) -> ("Current"=w381:u32)  [unwired: 1 in, 2 out]
                    n183 = property class="DigNum (strict)"(reference=w382, error in=w383, "Value"=w381) -> (error out=w384:errorcluster)  [unwired: 1 out]
                  }
                }
                n184 = property class="PmNumericParam`1[[System.Int64,"(reference=w358, error in=w354) -> (reference out=w356:refnum<k24>, error out=w353:errorcluster, "Available"=w357:bool)
                n185 = case shown="True" w357 {
                  tunnel: w356 -> [_ w379]
                  tunnel: w355 -> [_ w377]
                  tunnel: w353 -> [_ w376]
                  frame False {
                  }
                  frame True {
                    n186 = property class="PmNumericParam`1[[System.Int64,"(reference=w379, error in=w376) -> (error out=w375:errorcluster, "Current"=w378:i64)  [unwired: 1 out]
                    n187 = property class="DigNum (strict)"(reference=w377, error in=w375, "Value"=w378) -> ()  [unwired: 2 out]
                  }
                }
              }
            }
          }
          event "Scan Width": Value Change {
            w411 = 0 items=["Idle", "Capturing"] ("Status")
            n188 = event-data() -> ()  [unwired: 1 in, 6 out]
            n189 = property class="Camera"(reference=w405) -> (reference out=w404:refnum<k24>, "IsOpen"=w410:bool, "Status"=w412:i32)  [unwired: 1 in, 1 out]
            n190 = Equal?(x=w410, y=TRUE) -> (x = y?=w408:bool)
            n191 = Equal?(x=w412, y=w411) -> (x = y?=w407:bool)
            n192 = Equal?(x=w408, y=w407) -> (x = y?=w406:bool)
            n193 = control-ref of="Scan Line Time"() -> (w400:refnum<vi>)
            n194 = control-ref of="Scan Width"() -> (w402:refnum<vi>)
            n195 = control-ref of="Scan Line Delay"() -> (w401:refnum<vi>)
            n196 = case shown="True" w406 {
              tunnel: w404 -> [w413 w435]
              tunnel: [w413 w434] -> w403
              tunnel: w402 -> [_ w433]
              tunnel: w401 -> [_ w432]
              tunnel: w400 -> [_ w417]
              frame False {
              }
              frame True {
                n197 = property class="Camera"(reference=w435) -> (reference out=w434:refnum<k24>, "Settings"=w431:refnum<k24>)  [unwired: 1 in, 1 out]
                n198 = property class="CameraSettings"(reference=w431) -> (reference out=w414:refnum<k24>, error out=w427:errorcluster, "ScanWidth"=w430:refnum<k24>)  [unwired: 1 in]
                n199 = property class="PmNumericParam`1[[System.UInt32"(reference=w430, error in=w427) -> (reference out=w428:refnum<k24>, error out=w426:errorcluster, "Available"=w429:bool)
                n200 = case shown="True" w429 {
                  tunnel: w433 -> [_ w452]
                  tunnel: w428 -> [_ w451]
                  tunnel: w426 -> [w447 w450]
                  tunnel: [w447 w448] -> w422
                  frame False {
                  }
                  frame True {
                    n201 = property class="PmNumericParam`1[[System.UInt32"(reference=w451) -> (reference out=w455:refnum<k24>, "Max"=w453:u32, "Min"=w454:u32)  [unwired: 1 in, 1 out]
                    n202 = property class="DigNum (strict)"(reference=w452, error in=w450) -> (reference out=w459:refnum<vi>, error out=w449:errorcluster, "Value"=w458:dbl)
                    n203 = In Range and Coerce(upper limit=w453, x=w458, lower limit=w454) -> (coerced(x)=w457:dbl)  [unwired: 1 out]
                    n204 = property class="PmNumericParam`1[[System.UInt32"(reference=w455, "Current"=w457) -> (reference out=w456:refnum<k24>)  [unwired: 1 in, 1 out]
                    n205 = property class="PmNumericParam`1[[System.UInt32"(reference=w456) -> ("Current"=w460:u32)  [unwired: 1 in, 2 out]
                    n206 = property class="DigNum (strict)"(reference=w459, error in=w449, "Value"=w460) -> (error out=w448:errorcluster)  [unwired: 1 out]
                  }
                }
                n207 = property class="CameraSettings"(reference=w414) -> ("ScanLineDelay"=w421:refnum<k24>, "ScanLineTime"=w420:refnum<k24>)  [unwired: 1 in, 2 out]
                n208 = property class="PmNumericParam`1[[System.UInt32"(reference=w421, error in=w422) -> (reference out=w424:refnum<k24>, error out=w423:errorcluster, "Available"=w425:bool)
                n209 = case shown="True" w425 {
                  tunnel: w432 -> [_ w443]
                  tunnel: w424 -> [_ w446]
                  tunnel: w423 -> [w441 w444]
                  tunnel: [w441 w445] -> w416
                  frame False {
                  }
                  frame True {
                    n210 = property class="PmNumericParam`1[[System.UInt32"(reference=w446) -> ("Current"=w442:u32)  [unwired: 1 in, 2 out]
                    n211 = property class="DigNum (strict)"(reference=w443, error in=w444, "Value"=w442) -> (error out=w445:errorcluster)  [unwired: 1 out]
                  }
                }
                n212 = property class="PmNumericParam`1[[System.Int64,"(reference=w420, error in=w416) -> (reference out=w418:refnum<k24>, error out=w415:errorcluster, "Available"=w419:bool)
                n213 = case shown="True" w419 {
                  tunnel: w418 -> [_ w440]
                  tunnel: w417 -> [_ w438]
                  tunnel: w415 -> [_ w437]
                  frame False {
                  }
                  frame True {
                    n214 = property class="PmNumericParam`1[[System.Int64,"(reference=w440, error in=w437) -> (error out=w436:errorcluster, "Current"=w439:i64)  [unwired: 1 out]
                    n215 = property class="DigNum (strict)"(reference=w438, error in=w436, "Value"=w439) -> ()  [unwired: 2 out]
                  }
                }
              }
            }
          }
          event "Trigger In Behaviour", "Trigger Out Behaviour": Value Change {
            n216 = local read "Camera Status"() -> (w461:bool)
            n217 = event-data() -> ()  [unwired: 1 in, 6 out]
            n218 = case shown="True" w461 {
              tunnel: w464 -> [w466 w470]
              tunnel: [w466 w467] -> w463
              frame False {
                n219 = One Button Dialog(message="Camera is not open") -> ()  [unwired: 1 in, 1 out]
              }
              frame True {
                w475 = 0 items=["Idle", "Capturing"] ("Status")
                n220 = property class="Camera"(reference=w470) -> (reference out=w468:refnum<k24>, "IsOpen"=w474:bool, "Status"=w476:i32)  [unwired: 1 in, 1 out]
                n221 = Equal?(x=w474, y=TRUE) -> (x = y?=w472:bool)
                n222 = Equal?(x=w476, y=w475) -> (x = y?=w471:bool)
                n223 = Equal?(x=w472, y=w471) -> (x = y?=w469:bool)
                n224 = case shown="True" w469 {
                  tunnel: w468 -> [w477 w499]
                  tunnel: [w477 w491] -> w467
                  frame False {
                  }
                  frame True {
                    n225 = property class="Camera"(reference=w499) -> (reference out=w491:refnum<k24>, "Settings"=w486:refnum<k24>)  [unwired: 1 in, 1 out]
                    n226 = control-ref of="Trigger In Behaviour"() -> (w481:refnum<vi>)
                    n227 = control-ref of="Trigger Mode"() -> (w482:refnum<vi>)
                    n228 = control-ref of="Trigger Out Behaviour"() -> (w487:refnum<vi>)
                    n229 = control-ref of="Exp. out"() -> (w488:refnum<vi>)
                    n230 = property class="CameraSettings"(reference=w486) -> (reference out=w485:refnum<k24>, "ExposureTime"=w484:refnum<k24>, "ExposureMode"=w478:refnum<k24>, "ExposeOutMode"=w483:refnum<k24>)  [unwired: 1 in, 1 out]
                    n231 = property class="PmEnumParam"(reference=w483) -> (reference out=w489:refnum<k24>, "Available"=w490:bool)  [unwired: 1 in, 1 out]
                    n232 = property class="PmEnumParam"(reference=w478) -> (reference out=w480:refnum<k24>, "Available"=w479:bool)  [unwired: 1 in, 1 out]
                    n233 = property class="PmNumericParam`1[[System.UInt64"(reference=w484) -> (reference out=w496:refnum<k24>, "Max"=w498:u64, "Min"=w497:u64)  [unwired: 1 in, 1 out]
                    n234 = case shown="True" w490 {
                      tunnel: w489 -> [_ w524]
                      tunnel: w488 -> [_ w518]
                      tunnel: w487 -> [_ w515]
                      frame False {
                      }
                      frame True {
                        n235 = property class="CmbBox"(reference=w515) -> (reference out=w517:refnum<vi>, "Strings[]"=w525:string[])  [unwired: 1 in, 1 out]
                        n236 = property class="CmbBox"(reference=w517) -> ("Value"=w516:string)  [unwired: 1 in, 2 out]
                        n237 = while {
                          tunnel: w525 -> [w529] mode=indexing
                          tunnel: [w527] -> w522
                          tunnel: w516 -> [w526]
                          i -> [w527]
                          stop <- w528 stop-if-true
                          n238 = Equal?(x=w529, y=w526) -> (x = y?=w528:bool)
                        }
                        n239 = property class="PmEnumParam"(reference=w524) -> (reference out=w521:refnum<k24>, "Options"=w523:refnum<k24>)  [unwired: 1 in, 1 out]
                        n240 = invoke class="PmReadOnlyObservableCollection`" method="get_Item"(reference=w523, "index"=w522) -> ("get_Item"=w520:refnum<k24>)  [unwired: 2 in, 3 out]
                        n241 = property class="PmEnumItem"(reference=w520) -> ("Value"=w519:i32)  [unwired: 1 in, 2 out]
                        n242 = property class="PmEnumParam"(reference=w521, "Current"=w520) -> ()  [unwired: 1 in, 2 out]
                        n243 = property class="DigNum (strict)"(reference=w518, "Value"=w519) -> ()  [unwired: 1 in, 2 out]
                      }
                    }
                    n244 = case shown="True" w479 {
                      tunnel: w480 -> [_ w509]
                      tunnel: w482 -> [_ w503]
                      tunnel: w481 -> [_ w500]
                      frame False {
                      }
                      frame True {
                        n245 = property class="CmbBox"(reference=w500) -> (reference out=w502:refnum<vi>, "Strings[]"=w510:string[])  [unwired: 1 in, 1 out]
                        n246 = property class="CmbBox"(reference=w502) -> ("Value"=w501:string)  [unwired: 1 in, 2 out]
                        n247 = while {
                          tunnel: w510 -> [w514] mode=indexing
                          tunnel: [w512] -> w507
                          tunnel: w501 -> [w511]
                          i -> [w512]
                          stop <- w513 stop-if-true
                          n248 = Equal?(x=w514, y=w511) -> (x = y?=w513:bool)
                        }
                        n249 = property class="PmEnumParam"(reference=w509) -> (reference out=w506:refnum<k24>, "Options"=w508:refnum<k24>)  [unwired: 1 in, 1 out]
                        n250 = invoke class="PmReadOnlyObservableCollection`" method="get_Item"(reference=w508, "index"=w507) -> ("get_Item"=w505:refnum<k24>)  [unwired: 2 in, 3 out]
                        n251 = property class="PmEnumItem"(reference=w505) -> ("Value"=w504:i32)  [unwired: 1 in, 2 out]
                        n252 = property class="PmEnumParam"(reference=w506, "Current"=w505) -> ()  [unwired: 1 in, 2 out]
                        n253 = property class="DigNum (strict)"(reference=w503, "Value"=w504) -> ()  [unwired: 1 in, 2 out]
                      }
                    }
                    n254 = local read "Exposure Time"() -> (w493:dbl)
                    n255 = In Range and Coerce(upper limit=w498, x=w493, lower limit=w497) -> (coerced(x)=w494:dbl)  [unwired: 1 out]
                    n256 = property class="CameraSettings"(reference=w485, "Exposure"=w494) -> ()  [unwired: 1 in, 2 out]
                    n257 = property class="PmNumericParam`1[[System.UInt64"(reference=w496, "Current"=w494) -> (reference out=w495:refnum<k24>)  [unwired: 1 in, 1 out]
                    n258 = property class="PmNumericParam`1[[System.UInt64"(reference=w495) -> ("Current"=w492:u64)  [unwired: 1 in, 2 out]
                    n259 = local write "Exposure Time"(w492) -> ()
                  }
                }
              }
            }
          }
          event "Live start": Value Change {
            n260 = event-data() -> ()  [unwired: 1 in, 6 out]
            n261 = case shown="True" "Live start" {
              tunnel: w532 -> [w534 w537]
              tunnel: [w534 w536] -> w531
              frame False {
              }
              frame True {
                n262 = local read "Camera Status"() -> (w535:bool)
                n263 = case shown="True" w535 {
                  tunnel: w537 -> [w538 w543]
                  tunnel: [w538 w541] -> w536
                  frame False {
                    n264 = One Button Dialog(message="Camera is not open") -> ()  [unwired: 1 in, 1 out]
                  }
                  frame True {
                    w548 = 0 items=["Idle", "Capturing"] ("Status")
                    n265 = property class="Camera"(reference=w543) -> (reference out=w542:refnum<k24>, "IsOpen"=w547:bool, "Status"=w549:i32)  [unwired: 1 in, 1 out]
                    n266 = Equal?(x=w547, y=TRUE) -> (x = y?=w545:bool)
                    n267 = Equal?(x=w549, y=w548) -> (x = y?=w544:bool)
                    n268 = Equal?(x=w545, y=w544) -> (x = y?=w540:bool)
                    n269 = case shown="True" w540 {
                      tunnel: w542 -> [w551 w553]
                      tunnel: [w551 w554] -> w541
                      frame False {
                        n270 = local write "Live"(FALSE ("Live 2")) -> ()
                      }
                      frame True {
                        n271 = flat-sequence {
                          tunnel: w553 -> [w559]
                          tunnel: [w556] -> w552
                          frame #0 {
                            n272 = property class="Camera"(reference=w559) -> (reference out=w556:refnum<k24>, "AcquisitionBuffer"=w558:refnum<k24>)  [unwired: 1 in, 1 out]
                            n273 = property class="AcqBuffer"(reference=w558, "BufferSize"=100) -> ()  [unwired: 1 in, 2 out]
                          }
                        }
                        n274 = local write "Live"(TRUE ("Live")) -> ()
                        n275 = invoke class="Camera" method="StartLive"(reference=w552) -> (reference out=w554:refnum<k24>)  [unwired: 2 in, 2 out]
                      }
                    }
                  }
                }
              }
            }
          }
          event "Live stop": Value Change {
            n276 = event-data() -> ()  [unwired: 1 in, 6 out]
            n277 = case shown="True" "Live stop" {
              tunnel: w561 -> [w563 w566]
              tunnel: [w563 w565] -> w560
              frame False {
              }
              frame True {
                n278 = local read "Camera Status"() -> (w564:bool)
                n279 = case shown="False" w564 {
                  tunnel: w566 -> [w568 w578]
                  tunnel: [w568 w575] -> w565
                  frame False {
                    n280 = One Button Dialog(message="Camera is not open") -> ()  [unwired: 1 in, 1 out]
                  }
                  frame True {
                    w573 = 1 items=["Idle", "Capturing"] ("Status")
                    n281 = property class="Camera"(reference=w578) -> (reference out=w576:refnum<k24>, "IsOpen"=w572:bool, "Status"=w574:i32)  [unwired: 1 in, 1 out]
                    n282 = Equal?(x=w574, y=w573) -> (x = y?=w569:bool)
                    n283 = Equal?(x=w572, y=TRUE) -> (x = y?=w570:bool)
                    n284 = Equal?(x=w570, y=w569) -> (x = y?=w577:bool)
                    n285 = case shown="True" w577 {
                      tunnel: w576 -> [w579 w582]
                      tunnel: [w579 w581] -> w575
                      frame False {
                      }
                      frame True {
                        n286 = invoke class="Camera" method="Stop"(reference=w582) -> (reference out=w581:refnum<k24>)  [unwired: 2 in, 2 out]
                        n287 = local write "Live"(FALSE ("Live 2")) -> ()
                      }
                    }
                  }
                }
              }
            }
          }
          event "Uninit": Value Change {
            n288 = event-data() -> ()  [unwired: 1 in, 6 out]
            n289 = case shown="True" "Uninit" {
              tunnel: w587 -> [w589 w593]
              tunnel: [w589 w592] -> w586
              tunnel: [FALSE ("Camera Status") w590] -> w584
              frame False {
              }
              frame True {
                n290 = local read "Camera Status"() -> (w591:bool)
                n291 = case shown="True" w591 {
                  tunnel: w593 -> [w595 w600]
                  tunnel: [w595 w599] -> w592
                  tunnel: [FALSE ("Camera Status") w598] -> w590
                  frame False {
                  }
                  frame True {
                    n292 = local read "Live"() -> (w596:bool)
                    n293 = Not(x=w596) -> (.not. x?=w597:bool)
                    n294 = case shown="True" w597 {
                      tunnel: w600 -> [w602 w605]
                      tunnel: [w602 w604] -> w599
                      tunnel: [FALSE ("Camera Status") w603] -> w598
                      frame False {
                      }
                      frame True {
                        n295 = flat-sequence {
                          tunnel: w605 -> [w608]
                          tunnel: [w607] -> w606
                          tunnel: [w611] -> w604
                          tunnel: w606 -> [w611]
                          tunnel: [TRUE ("Camera Status")] -> w603
                          frame #0 {
                            n296 = invoke class="Camera" method="Close"(reference=w608) -> (reference out=w607:refnum<k24>)  [unwired: 2 in, 2 out]
                          }
                          frame #1 {
                            n297 = local write "Camera Status"(FALSE ("Camera Status")) -> ()
                          }
                        }
                      }
                    }
                  }
                }
              }
            }
          }
        }
      }
    }
    frame #2 {
      n298 = invoke class="Library" method="Release"(reference=w613) -> (reference out=w614:refnum<k24>)  [unwired: 2 in, 2 out]
      n299 = Wait (ms)(milliseconds to wait=u32 100) -> ()  [unwired: 1 out]
      n300 = Close Reference(reference=w614) -> ()  [unwired: 1 in, 1 out]
    }
    frame #3 {
      n301 = invoke class="GC" method="Collect"() -> ()  [unwired: 3 in, 3 out]
    }
  }
  n302 = control-ref of="Exp. out"() -> (w3:refnum<vi>)
  n303 = property class="DigNum (strict)"(reference=w3, "Visible"=FALSE) -> ()  [unwired: 1 in, 2 out]
  n304 = control-ref of="Trigger Mode"() -> (w2:refnum<vi>)
  n305 = property class="DigNum (strict)"(reference=w2, "Visible"=FALSE) -> ()  [unwired: 1 in, 2 out]
  n306 = control-ref of="Trigger Out Behaviour"() -> (w8:refnum<vi>)
  n307 = control-ref of="Exp. out"() -> (w6:refnum<vi>)
  n308 = property class="DigNum (strict)"(reference=w6, "Value"=0) -> ()  [unwired: 1 in, 2 out]
  n309 = property class="CmbBox"(reference=w8, "Value"="") -> ()  [unwired: 1 in, 2 out]
  n310 = local write "Camera Status"(FALSE ("Camera Status")) -> ()
  n311 = property on="Scan Width" class="DigNum (strict)"("DisabledEnum"=w11) -> ()  [unwired: 2 in, 2 out]
  n312 = property on="Scan Line Delay" class="DigNum (strict)"("DisabledEnum"=w11) -> ()  [unwired: 2 in, 2 out]
  n313 = control-ref of="Scan Line Delay"() -> (w14:refnum<vi>)
  n314 = control-ref of="Scan Width"() -> (w17:refnum<vi>)
  n315 = control-ref of="Scan Line Time"() -> (w13:refnum<vi>)
  n316 = control-ref of="Scan Direction"() -> (w20:refnum<vi>)
  n317 = control-ref of="Scan Mode"() -> (w23:refnum<vi>)
  n318 = property class="CmbBox"(reference=w23, "Value"="", "Strings[]"=string[] [] ("Strings []")) -> ()  [unwired: 1 in, 2 out]
  n319 = property class="DigNum (strict)"(reference=w14, "Value"=0.0) -> ()  [unwired: 1 in, 2 out]
  n320 = property class="CmbBox"(reference=w20, "Strings[]"=string[] [] ("Strings []"), "Value"="") -> ()  [unwired: 1 in, 2 out]
  n321 = property class="DigNum (strict)"(reference=w17, "Value"=0.0) -> ()  [unwired: 1 in, 2 out]
  n322 = property class="DigNum (strict)"(reference=w13, "Value"=0.0) -> ()  [unwired: 1 in, 2 out]
  n323 = local write "Scan Direction Reset"(FALSE ("Boolean")) -> ()
  "Boolean" <- FALSE ("Boolean")
